vi "create_target_abs.vi"(11 "Inputs":dbl[](array[numeric])) -> (3 "Target Array":dbl[](array[numeric]))   [LabVIEW 2015]
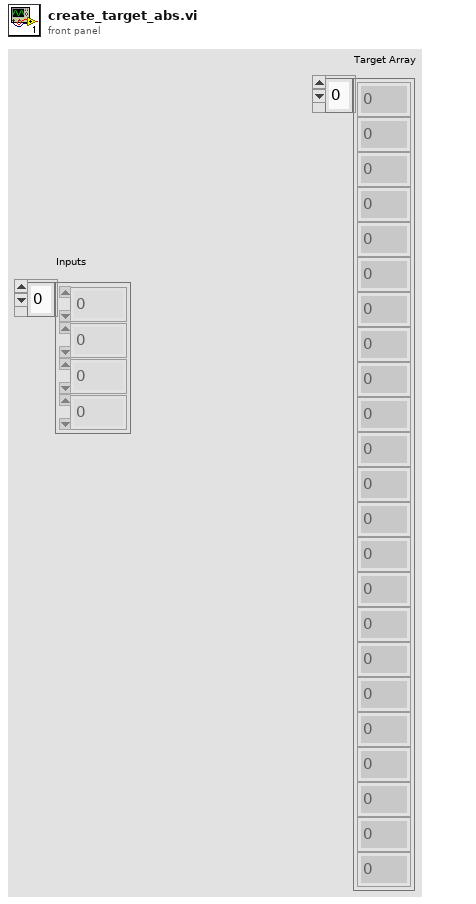
[diagram p1: front panel]
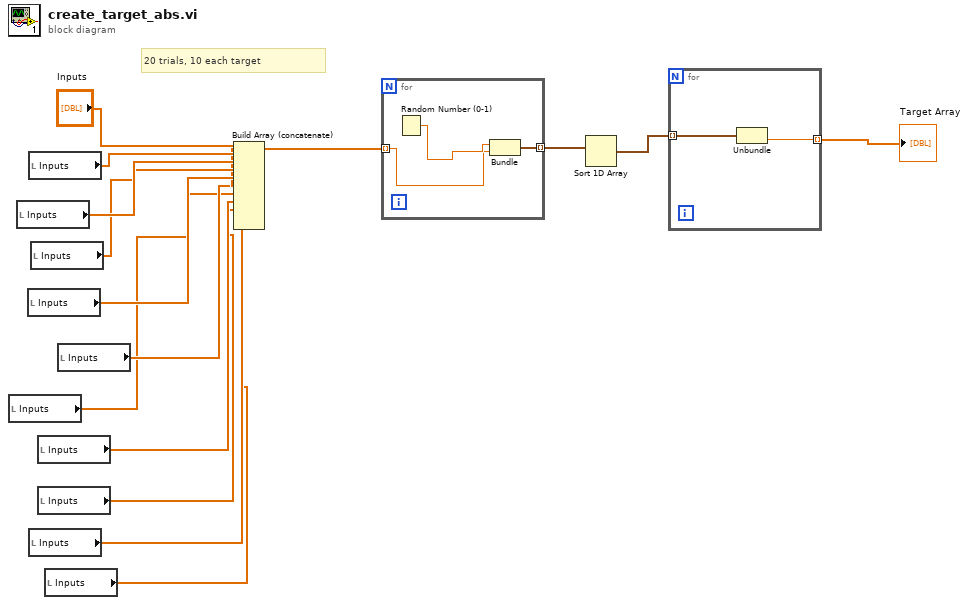
[diagram p0: block diagram]
diagram:
  # "20 trials, 10 each target"
  n1 = local read "Inputs"() -> (w5:dbl[])
  n2 = local read "Inputs"() -> (w10:dbl[])
  n3 = local read "Inputs"() -> (w8:dbl[])
  n4 = local read "Inputs"() -> (w11:dbl[])
  n5 = local read "Inputs"() -> (w2:dbl[])
  n6 = local read "Inputs"() -> (w9:dbl[])
  n7 = local read "Inputs"() -> (w4:dbl[])
  n8 = local read "Inputs"() -> (w3:dbl[])
  n9 = local read "Inputs"() -> (w1:dbl[])
  n10 = local read "Inputs"() -> (w6:dbl[])
  n11 = Build Array (concatenate)("Inputs", w11, w10, w9, w8, w6, w5, w4, w3, w2, w1) -> (w7:dbl[])
  n12 = for {
    tunnel: w7 -> [w17] mode=indexing
    tunnel: [w16] -> w14 mode=indexing
    n13 = Random Number (0-1)() -> (number: 0 to 1=w18:dbl)
    n14 = Bundle("number: 0 to 1"=w18, "Numeric"=w17) -> (w16:cluster{"number: 0 to 1":dbl, "Numeric":dbl})  [unwired: 1 in]
  }
  n15 = Sort 1D Array(array=w14) -> (sorted array=w15:cluster{"number: 0 to 1":dbl, "Numeric":dbl}[])
  n16 = for {
    tunnel: w15 -> [w20] mode=indexing
    tunnel: [w19] -> w13 mode=indexing
    n17 = Unbundle(w20) -> ("Numeric"=w19:dbl)  [unwired: 1 out]
  }
  "Target Array" <- w13
